vi "ALTS-2015 DB Serial Details Driver.vi"(0 "Serial Number":string, 1 "Operation":T2=enum."Read DB", 11 "error in (no error)":errorcluster) -> (4 "S No Valid?":bool, 8 "Serial Details from DB":T1, 15 "error out":errorcluster)   [LabVIEW 2013]
doc: "Copyright © 2005, Soliton Technologies.\nAll rights reserved."
uses:
  Controls/ALTS-2015 DB Driver Options.ctl
  Controls/ALTS-2015 Serial DB Details.ctl
  <vilib>/addons/database/Auxilliary.llb/DB Tools Parameter Info.ctl
  <vilib>/addons/database/Auxilliary.llb/DB Tools DataTypes.ctl
  <vilib>/addons/database/Auxilliary.llb/DB Tools Parameter Dir.ctl
  Controls/ALTS-2015 LV2GBL Options.ctl
  <vilib>/addons/database/Command.llb/Cmd ObjectReference.ctl
  <vilib>/addons/database/Connection.llb/DB Tools Open Connec (Path).vi
  <vilib>/addons/database/Command.llb/Cmd Set Parameter Value (C).vi
  <vilib>/addons/database/Command.llb/Cmd Execute.vi
  <vilib>/addons/database/Recordset.llb/Rec Fetch Recordset Data (R).vi
  <vilib>/addons/database/Recordset.llb/Rec Destroy - Connection.vi
  <vilib>/Utility/file.llb/Read From Spreadsheet File (string).vi
  <vilib>/addons/database/Command.llb/Cmd Delete.vi
  <vilib>/addons/database/_DB Variant To Data/Database Variant To Data.xnode
  <vilib>/addons/database/NI_Database_API.lvlib
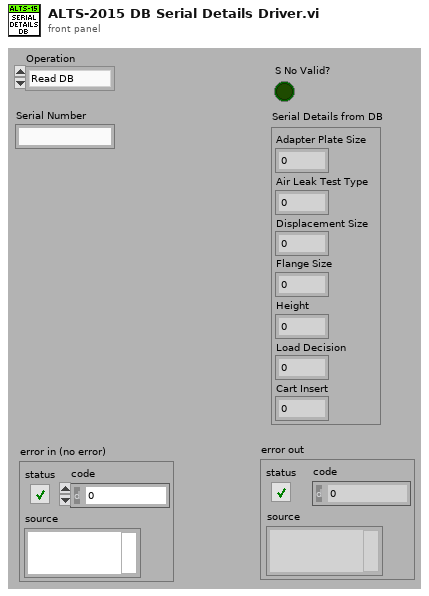
[diagram p1: front panel]
types:
  T1 = typedef "ALTS-2015 Serial DB Details.ctl" = cluster{"Adapter Plate Size":i32, "Air Leak Test Type ":i32, "Displacement Size":i32, "Flange Size":i32, "Height":i32, "Load Decision":i32, "Cart Insert":i32}
  T2 = typedef "ALTS-2015 DB Driver Options.ctl" = enum16{"Init", "Read DB", "Close"}
  T3 = typedef "ALTS-2015 LV2GBL Options.ctl" = enum16{"Read all", "Write all"}
  T4 = typedef "NI_Database_API.lvlib/DB Tools Parameter Info.ctl" = cluster{"parameter name":string, "type":T5, "direction":T6, "value":variant}
  T5 = typedef "NI_Database_API.lvlib/DB Tools DataTypes.ctl" = enum16{"String", "Long (I32)", "Single (SGL)", "Double (DBL)", "Date/Time", "Binary"}
  T6 = typedef "NI_Database_API.lvlib/DB Tools Parameter Dir.ctl" = enum32{"Input", "Output", "Input/Output", "Return Value"}
  T7 = typedef "ALTS-2015 INI Configuration Cluster.ctl" = cluster{"Application":cluster{"Rerun Count":i32, "Workorder No":string, "PLC Scanner":bool}, "Station Details":cluster{"Sensor Name 1":string, "Sensor Name 2":string, "Sensor Name 3":string, "Sensor Name 4":string, "Station1 Enable":bool, "Station2 Enable":bool, "Station3 Enable":bool, "Station4 Enable":bool}, "Database":cluster{"Database Connection Link":path, "Result Procedure":string, "User":string, "Password":string, "Prompt":bool, "Station 1 LT Result DB DSN Path":path, "Station 2 LT Result DB DSN Path":path, "Station 3 LT Result DB DSN Path":path, "Station 4 LT Result DB DSN Path":path, "AirLeakTestResult Procedure":string, "Serial Details Procedure":string}, "Simulation":cluster{"Simulate DAQ Hardware":bool, "Simulate Result DB Write":bool, "Simulate Scanner":bool, "Simulate OPC":bool, "Simulate Serial Details DB":bool, "Simulate Result DB":bool, "Simulate Scanner DB Path":path, "Simulate Serial Details DB Path":path, "Simulate Result DB Path":path}, "Barcode Scanner1":cluster{"Scanner IP":string, "Scanner Port":u16, "#Bytes to Read":i32, "Timeout_ms":i32}, "Barcode Scanner2":cluster{"Enabled?":bool, "Scanner IP":string, "Scanner Port":u16, "#Bytes to Read":i32}}
  T8 = typedef "NI_Database_API.lvlib/Conn ObjectReference.ctl" = refnum<k1>
  T9 = typedef "NI_Database_API.lvlib/Cmd ObjectReference.ctl" = refnum<k1>
  T10 = typedef "NI_Database_API.lvlib/Cmd-Rec Object Reference.ctl" = refnum<k1>
  T11 = typedef "NI_Database_API.lvlib/Cmd-Rec Data Members.ctl" = cluster{"recordset reference":T12, "command reference":T9}
  T12 = typedef "NI_Database_API.lvlib/Rec ObjectReference.ctl" = refnum<k1>
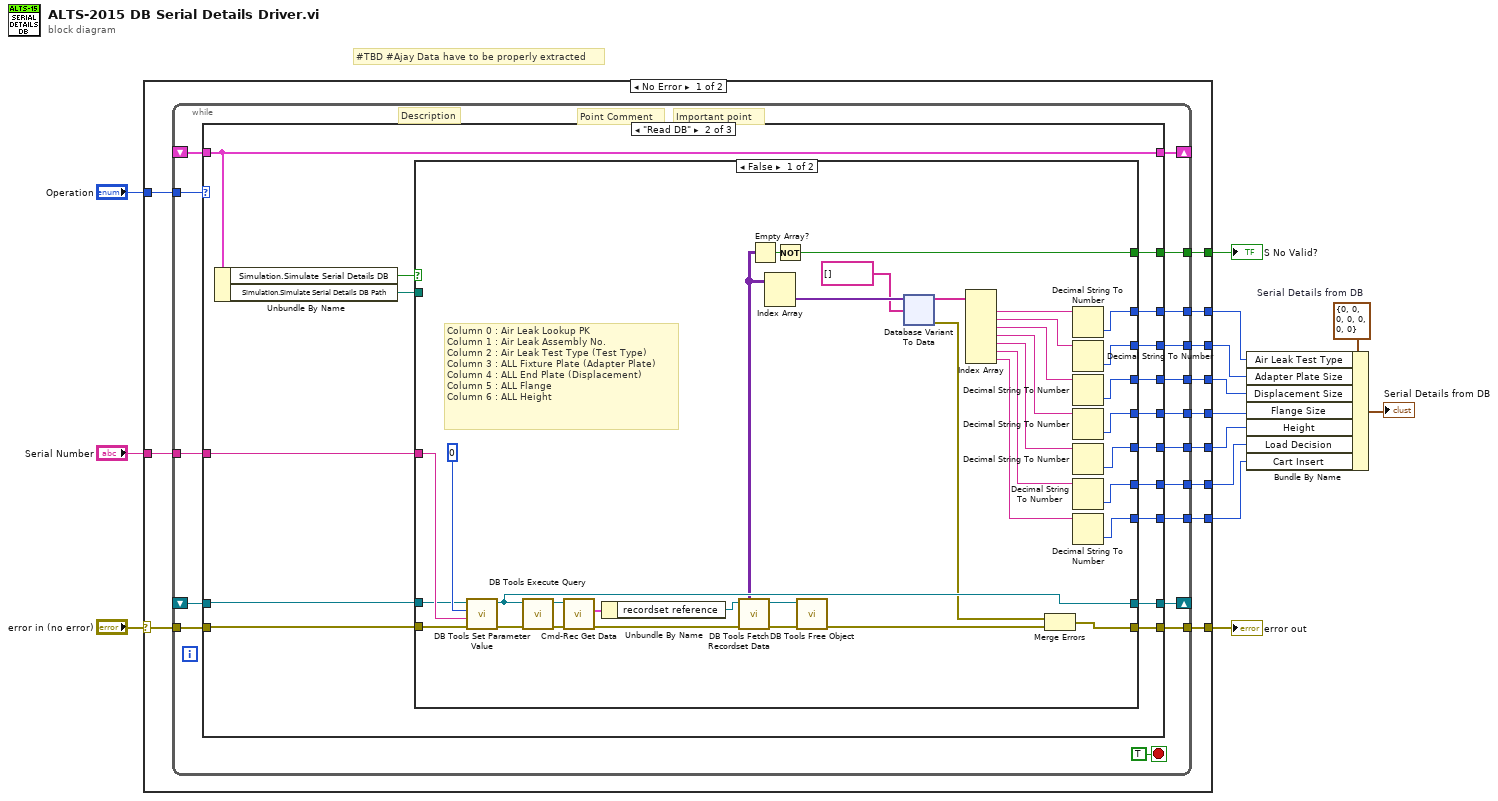
[diagram p0: block diagram]
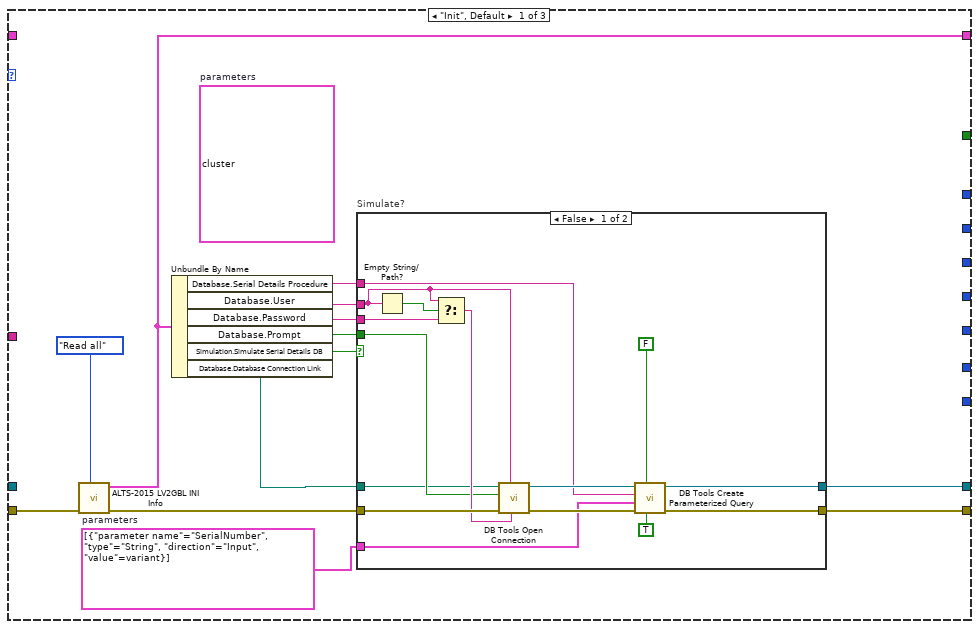
[diagram p2: hidden frame]
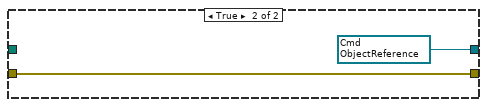
[diagram p3: hidden frame]
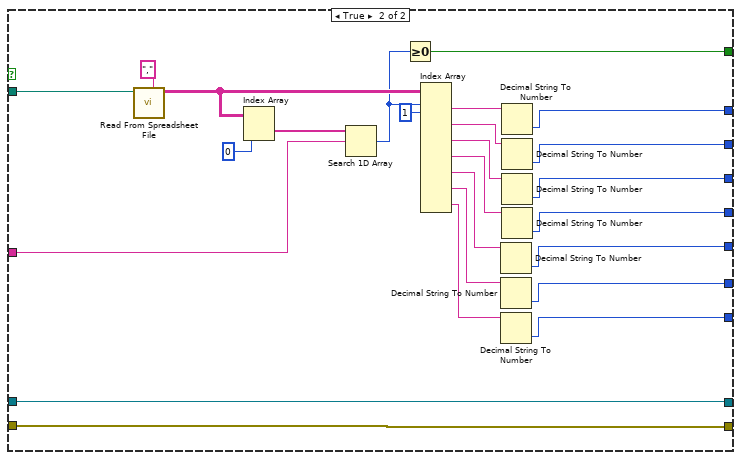
[diagram p4: hidden frame]
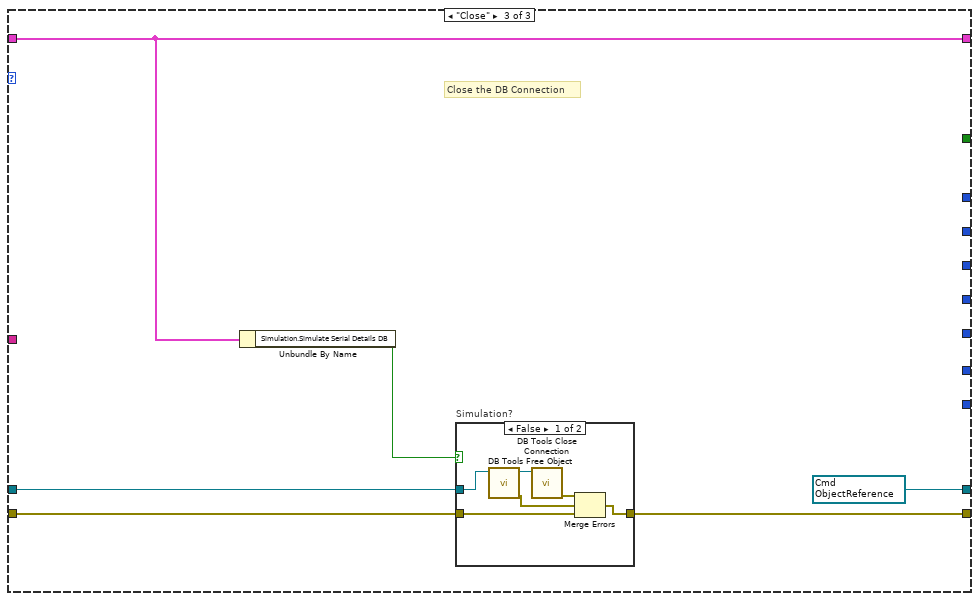
[diagram p5: hidden frame]
diagram:
  w8 = T1 {"Adapter Plate Size"=0, "Air Leak Test Type "=0, "Displacement Size"=0, "Flange Size"=0, "Height"=0, "Load Decision"=0, "Cart Insert"=0}  # Serial Details from DB
  # "#TBD #Ajay Data have to be properly extracted"
  n1 = case shown="No Error" "error in (no error)" {
    selector: "error in (no error)" -> [w25 w202]
    tunnel: [w26 w202] -> w13
    tunnel: "Operation" -> [w24 _]
    tunnel: "Serial Number" -> [w23 _]
    tunnel: [w22 _] -> w10
    tunnel: [w21 _] -> w4
    tunnel: [w20 _] -> w3
    tunnel: [w19 _] -> w1
    tunnel: [w18 _] -> w2
    tunnel: [w17 _] -> w5
    tunnel: [w16 _] -> w6
    tunnel: [w15 _] -> w7
    frame No Error {
      # "Point Comment"
      # "Important point"
      # "Description"
      n2 = while {
        tunnel: [w42] -> w26
        shift-right: [w41] -> _
        shift-left: _ -> [w40]
        tunnel: w25 -> [w39]
        tunnel: w24 -> [w38]
        tunnel: w23 -> [w37]
        tunnel: [w36] -> w22
        shift-right: [w35] -> _
        shift-left: _ -> [w34]
        tunnel: [w33] -> w21
        tunnel: [w32] -> w20
        tunnel: [w31] -> w19
        tunnel: [w30] -> w18
        tunnel: [w29] -> w17
        tunnel: [w28] -> w16
        tunnel: [w27] -> w15
        stop <- TRUE stop-if-true
        n3 = case shown="\"Read DB\"" w38 {
          tunnel: w39 -> [w48 w88 w191]
          tunnel: [w56 w89 w194] -> w42
          tunnel: [w55 w86 w189] -> w41
          tunnel: w40 -> [_ w87 w193]
          tunnel: w37 -> [_ w85 _]
          tunnel: [_ w82 _] -> w36
          tunnel: [w46 w81 w190] -> w35
          tunnel: w34 -> [_ w81 w190]
          tunnel: [_ w80 _] -> w33
          tunnel: [_ w79 _] -> w32
          tunnel: [_ w78 _] -> w31
          tunnel: [_ w77 _] -> w30
          tunnel: [_ w76 _] -> w29
          tunnel: [_ w75 _] -> w28
          tunnel: [_ w74 _] -> w27
          frame "Init", Default {
            (unwired) T4[] [{"parameter name"="ALL_AirLeakTest", "type"=enum."String", "direction"=enum."Output", "value"=variant}, {"parameter name"="ALL_FixturePlate", "type"=enum."String", "direction"=enum."Output", "value"=variant}, {"parameter name"="ALL_EndSize", "type"=enum."String", "direction"=enum."Output", "value"=variant}, {"parameter name"="ALL_Flange", "type"=enum."String", "direction"=enum."Output", "value"=variant}, {"parameter name"="ALL_Height", "type"=enum."String", "direction"=enum."Output", "value"=variant}, {"parameter name"="ALL_LoadDecision", "type"=enum."String", "direction"=enum."Output", "value"=variant}, {"parameter name"="ALL_CartInsert", "type"=enum."String", "direction"=enum."Output", "value"=variant}]  # parameters
            w44 = T4[] [{"parameter name"="SerialNumber", "type"=enum."String", "direction"=enum."Input", "value"=variant}]  # parameters
            n4 = call "ALTS-2015 LV2GBL INI Info.vi"("Options"=ALTS-2015_LV2GBL_Options."Read all", "error in"=w48) -> ("error out"=w47:errorcluster, "Configuration Cluster Out"=w46:T7)  [unwired: 8 in]
            n5 = Unbundle By Name(w46) -> ("Database.Serial Details Procedure"=w49:string, "Database.User"=w52:string, "Database.Password"=w51:string, "Database.Prompt"=w50:bool, "Simulation.Simulate Serial Details DB"=w53:bool, "Database.Database Connection Link"=w54:path)
            n6 = case "Simulate?" shown="False" w53 {
              tunnel: [w60 w73] -> w56
              tunnel: [w61 w72] -> w55
              tunnel: w54 -> [w57 _]
              tunnel: w47 -> [w71 w73]
              tunnel: w52 -> [w68 _]
              tunnel: w51 -> [w67 _]
              tunnel: w50 -> [w66 _]
              tunnel: w49 -> [w63 _]
              tunnel: w44 -> [w58 _]
              frame False {
                n7 = Empty String/Path?(string/path=w68) -> (empty?=w70:bool)
                n8 = Select(t=w68, s=w70, f=w67) -> (s? t:f=w69:string)
                n9 = call-poly <vilib>:"DB Tools Open Connection.vi"("password"=w69, "userID"=w68, "error in (no error)"=w71, "prompt? (F)"=w66, "connection information"=w57) -> ("error out"=w59:errorcluster, "connection reference"=w64:T8)  [unwired: 3 in]
                n10 = call <vilib>:"DB Tools Create Parameterized Query.vi"("stored procedure? (F)"=TRUE ("stored procedure? (f)"), "auto-detect parameters? (F)"=FALSE ("auto-detect parameters? (f)"), "error in (no error)"=w59, "parameters"=w58, "SQL query"=w63, "connection reference"=w64) -> ("error out"=w60:errorcluster, "command reference"=w61:T9)  [unwired: 1 in, 1 out]
              }
              frame True {
                w72 = T9 refnum items=["Command"] ("command reference")
              }
            }
          }
          frame "Read DB" {
            n11 = Unbundle By Name(w81) -> ("Simulation.Simulate Serial Details DB"=w84:bool, "Simulation.Simulate Serial Details DB Path"=w83:path)
            n12 = case shown="False" w84 {
              tunnel: [w97 w188] -> w89
              tunnel: w88 -> [w119 w188]
              tunnel: w87 -> [w120 w187]
              tunnel: [w112 w187] -> w86
              tunnel: w85 -> [w123 w182]
              tunnel: w83 -> [_ w186]
              tunnel: [w111 w177] -> w82
              tunnel: [w99 w166] -> w80
              tunnel: [w104 w172] -> w79
              tunnel: [w106 w176] -> w78
              tunnel: [w105 w171] -> w77
              tunnel: [w103 w170] -> w76
              tunnel: [w101 w164] -> w75
              tunnel: [w100 w165] -> w74
              frame False {
                # "Column 0 : Air Leak Lookup PK\nColumn 1 : Air Leak Assembly No.\nColumn 2 : Air Leak Test Type (Test Type)\nColumn 3 : ALL Fixture Plate (Adapter Plate)\nColumn 4 : ALL End Plate (Displacement)\nColumn 5 : ALL Flange\nColumn 6 : ALL Height"
                n13 = call-poly <vilib>:"DB Tools Set Parameter Value.vi"("error in (no error)"=w119, "value"=w123, "parameter index"=0, "command reference"=w120) -> ("error out"=w118:errorcluster, "command reference out"=w112:T9)  [unwired: 4 in]
                n14 = call-poly <vilib>:"DB Tools Execute Query.vi"("error in (no error)"=w118, "command reference"=w112) -> ("error out"=w114:errorcluster, "command-recordset reference"=w115:T10)  [unwired: 6 in]
                n15 = call <vilib>:"Cmd-Rec Get Data.vi"("error in (no error)"=w114, "command-recordset reference"=w115) -> ("error out"=w113:errorcluster, "data"=w117:T11)  [unwired: 2 in, 2 out]
                n16 = Unbundle By Name(w117) -> ("recordset reference"=w116:T12)
                n17 = call-poly <vilib>:"DB Tools Fetch Recordset Data.vi"("error in (no error)"=w113, "recordset reference"=w116) -> ("error out"=w121:errorcluster, "recordset data"=w110:variant[][], "recordset reference out"=w124:T12)  [unwired: 3 in]
                n18 = Empty Array?(array=w110) -> (empty?=w122:bool)
                n19 = Index Array(array=w110) -> (element=w109:variant[])  [unwired: 2 in]
                n20 = Not(x=w122) -> (.not. x?=w111:bool)
                n21 = call-poly <vilib>:"DB Tools Free Object.vi"("error in (no error)"=w121, "recordset reference"=w124) -> ("error out"=w98:errorcluster)  [unwired: 8 in, 1 out]
                n22 = xnode "Database Variant To Data"("database variant"=w109, "type"=string[] []) -> ("data"=w108:string[], "error out"=w96:errorcluster)  [unwired: 1 in]
                n23 = Index Array(array=w108) -> (element #1=w107:string, element #2=w95:string, element #3=w94:string, element #4=w93:string, element #5=w92:string, element #6=w91:string, element #7=w90:string)  [unwired: 7 in]
                n24 = Merge Errors(w96, w98) -> (w97:errorcluster)
                n25 = Decimal String To Number(string=w107) -> (number=w106:i32)  [unwired: 2 in, 1 out]
                n26 = Decimal String To Number(string=w95) -> (number=w105:i32)  [unwired: 2 in, 1 out]
                n27 = Decimal String To Number(string=w94) -> (number=w104:i32)  [unwired: 2 in, 1 out]
                n28 = Decimal String To Number(string=w93) -> (number=w99:i32)  [unwired: 2 in, 1 out]
                n29 = Decimal String To Number(string=w92) -> (number=w103:i32)  [unwired: 2 in, 1 out]
                n30 = Decimal String To Number(string=w91) -> (number=w101:i32)  [unwired: 2 in, 1 out]
                n31 = Decimal String To Number(string=w90) -> (number=w100:i32)  [unwired: 2 in, 1 out]
              }
              frame True {
                n32 = call-poly <vilib>:"Read From Spreadsheet File.vi"("delimiter (\\t)"="," ("delimiter (\\t)"), "file path (dialog if empty)"=w186) -> ("all rows"=w181:string[][])  [unwired: 5 in, 4 out]
                n33 = Index Array(array=w181, index (col)=0 ("disabled index (col)")) -> (element=w183:string[])  [unwired: 1 in]
                n34 = Search 1D Array(1D array=w183, element=w182) -> (index of element=w178:i32)  [unwired: 1 in]
                n35 = Greater Or Equal To 0?(x=w178) -> (x >= 0?=w177:bool)
                n36 = Index Array(array=w181, index (row) #1=w178, index (col) #1=1 ("disabled index (col)")) -> (element #1=w179:string, element #2=w175:string, element #3=w174:string, element #4=w173:string, element #5=w169:string, element #6=w168:string, element #7=w167:string)  [unwired: 12 in]
                n37 = Decimal String To Number(string=w169) -> (number=w170:i32)  [unwired: 2 in, 1 out]
                n38 = Decimal String To Number(string=w168) -> (number=w164:i32)  [unwired: 2 in, 1 out]
                n39 = Decimal String To Number(string=w167) -> (number=w165:i32)  [unwired: 2 in, 1 out]
                n40 = Decimal String To Number(string=w179) -> (number=w176:i32)  [unwired: 2 in, 1 out]
                n41 = Decimal String To Number(string=w175) -> (number=w171:i32)  [unwired: 2 in, 1 out]
                n42 = Decimal String To Number(string=w174) -> (number=w172:i32)  [unwired: 2 in, 1 out]
                n43 = Decimal String To Number(string=w173) -> (number=w166:i32)  [unwired: 2 in, 1 out]
              }
            }
          }
          frame "Close" {
            w189 = T9 refnum items=["Command"] ("command reference")
            # "Close the DB Connection"
            n44 = Unbundle By Name(w190) -> ("Simulation.Simulate Serial Details DB"=w192:bool)
            n45 = case "Simulation?" shown="False" w192 {
              tunnel: [w195 w201] -> w194
              tunnel: w193 -> [w200 _]
              tunnel: w191 -> [w196 w201]
              frame False {
                n46 = call-poly <vilib>:"DB Tools Free Object.vi"("command reference"=w200) -> ("error out"=w197:errorcluster, "connection reference"=w199:T8)  [unwired: 9 in]
                n47 = call <vilib>:"DB Tools Close Connection.vi"("connection reference"=w199) -> ("error out"=w198:errorcluster)  [unwired: 6 in]
                n48 = Merge Errors(w198, w197, w196) -> (w195:errorcluster)
              }
              frame True {
              }
            }
          }
        }
      }
    }
    frame Error {
    }
  }
  "error out" <- w13
  "S No Valid?" <- w10
  n49 = Bundle By Name(cluster=w8, "Air Leak Test Type"=w1, "Adapter Plate Size"=w2, "Displacement Size"=w3, "Flange Size"=w4, "Height"=w5, "Load Decision"=w6, "Cart Insert"=w7) -> (→"Serial Details from DB":T1)
